vi "Configure Burst Count [BST] Core.vi"(8 "error in (no error)":errorcluster, 9 "burst count (1)":i32=1, 10 "Channel Name (\"\")":string="CHANNEL1" caption="channel name (\"CHANNEL1\")", 11 "IVI_Fgen in":refnum<class "IVI_Fgen.lvclass">) -> (0 "error out":errorcluster, 3 "IVI_Fgen out":refnum<class "IVI_Fgen.lvclass">)   [LabVIEW 2013, in "IVI_Fgen.lvlib" / "IVI_Fgen.lvclass"]
doc: "This VI configures the burst count. When the function generator receives a trigger while in the Burst operation mode, it generates the number of waveform cycles you specify in the Count control.\n\nNotes:\n\n(1) This VI is part of the IviFgenBurst [BST] extension group."
uses:
  IVI_Fgen.lvclass
  IVI_Fgen.lvclass/IVI_Fgen.ctl
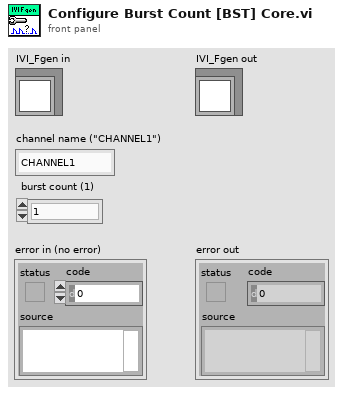
[diagram p1: front panel]
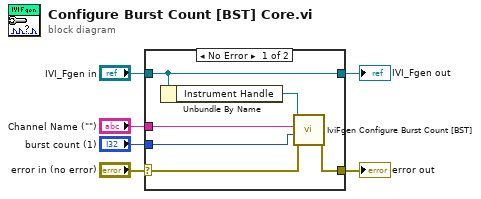
[diagram p0: block diagram]
diagram:
  n1 = case shown="No Error" "error in (no error)" {
    selector: "error in (no error)" -> [w10 w14]
    tunnel: [w9 w14] -> w5
    tunnel: [w12 w13] -> w3
    tunnel: "IVI_Fgen in" -> [w12 w13]
    tunnel: "Channel Name (\"\")" -> [w8 _]
    tunnel: "burst count (1)" -> [w7 _]
    frame No Error {
      n2 = Unbundle By Name(w12) -> ("Instrument Handle"=w11:refnum<k15>)
      n3 = call <vilib>:"IviFgen Configure Burst Count [BST].vi"("error in (no error)"=w10, "burst count (1)"=w7, "channel name (\"CHANNEL1\")"=w8, "instrument handle"=w11) -> ("error out"=w9:errorcluster)  [unwired: 6 in, 1 out]
    }
    frame Error {
    }
  }
  "error out" <- w5
  "IVI_Fgen out" <- w3
